vi "Open Panels in Device List.vi"(7 "Index Value":u32, 8 "error in (no error)":errorcluster, 9 "Subpanels to open":bool[](array[boolean]), 10 "Active List":u16[](array[numeric]), 11 "Device List State":T1) -> (0 "error out":errorcluster, 3 "Device List State out":T1)   [LabVIEW 2015]
uses:
  Device List State.ctl
  Device/Device.lvclass
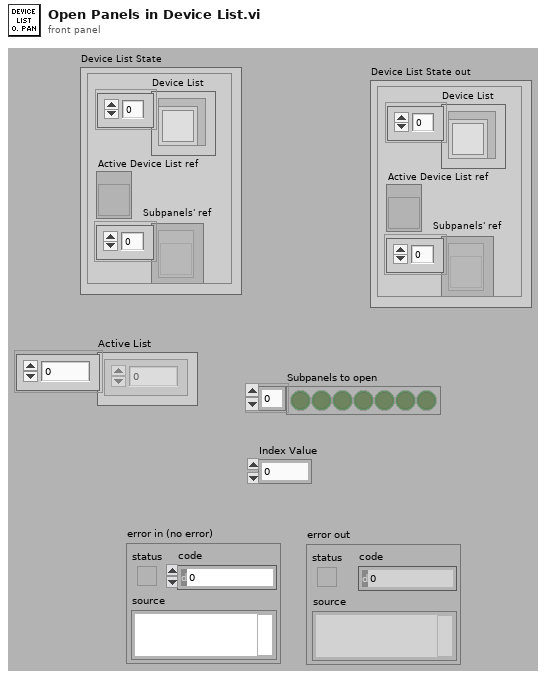
[diagram p1: front panel]
types:
  T1 = typedef "Device List State.ctl" = cluster{"Device List":refnum<class "Device.lvclass">[], "Active Device List ref":refnum<vi>, "Subpanels' ref":refnum<vi>[]}
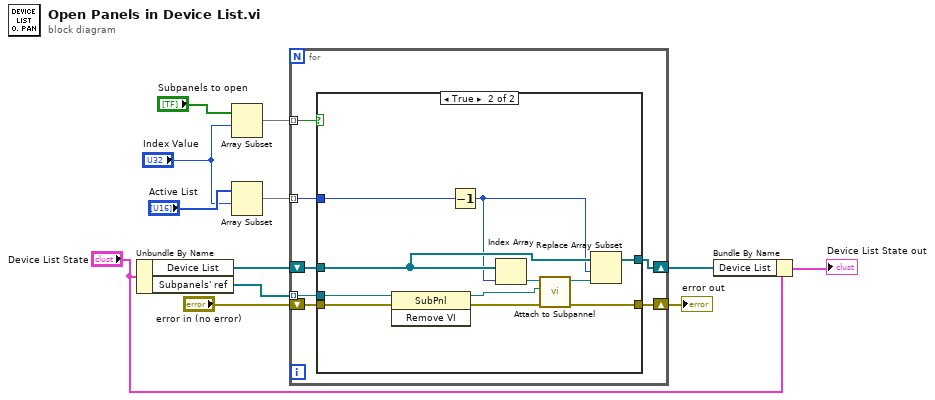
[diagram p0: block diagram]
diagram:
  n1 = Unbundle By Name("Device List State") -> ("Device List"=w5:refnum<class "Device.lvclass">[], "Subpanels' ref"=w4:refnum<vi>[])
  n2 = Array Subset(array="Subpanels to open", index="Index Value") -> (w12:bool[])  [unwired: 1 in]
  n3 = Array Subset(array="Active List", index="Index Value") -> (w11:u16[])  [unwired: 1 in]
  n4 = for {
    tunnel: w4 -> [w18] mode=indexing
    tunnel: w12 -> [w19] mode=indexing
    shift-right: [w16] -> w6
    shift-left: "error in (no error)" -> [w17]
    tunnel: w11 -> [w15] mode=indexing
    shift-right: [w13] -> w2
    shift-left: w5 -> [w14]
    n5 = case shown="True" w19 {
      tunnel: w18 -> [_ w32]
      tunnel: w17 -> [w21 w24]
      tunnel: [w21 w26] -> w16
      tunnel: w15 -> [_ w22]
      tunnel: w14 -> [w20 w30]
      tunnel: [w20 w27] -> w13
      frame False {
      }
      frame True {
        n6 = invoke class="SubPnl" method="Remove VI"(reference=w32, error in=w24) -> (reference out=w25:refnum<vi>, error out=w23:errorcluster)  [unwired: 1 in, 1 out]
        n7 = Decrement(x=w22) -> (x-1=w29:u16)
        n8 = Index Array(array=w30, index=w29) -> (element=w31:refnum<class "Device.lvclass">)
        n9 = call "Attach to Subpannel.vi"("error in (no error)"=w23, "Sub Panel"=w25, "Device in"=w31) -> ("error out"=w26:errorcluster, "Device out"=w28:refnum<class "Device.lvclass">)  [unwired: 7 in]
        n10 = Replace Array Subset(array=w30, new element=w28, index=w29) -> (w27:refnum<class "Device.lvclass">[])
      }
    }
  }
  "error out" <- w6
  n11 = Bundle By Name(cluster="Device List State", "Device List"=w2) -> (→"Device List State out":T1)
